vi "TalonWorking.vi"(1 "Name":string) -> (0 "Broken":bool)   [LabVIEW 2017]
uses:
  <vilib>/Rock Robotics/Network Tables/NT Write Boolean.vi
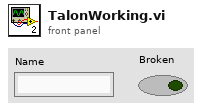
[diagram p1: front panel]
types:
  T1 = typedef "WPI_MotorControlDeviceRef.ctl" = cluster{"DeviceStatus":errorcluster, "Type":T2, "PWM":cluster{"PWM Channel":T3, "DeadBand":T4}, "CAN":cluster{"Device Number":u8, "SetOutput VI Ref":variant, "GetOutput VI Ref":variant, "Enable VI Ref":variant, "Disable VI Ref":variant, "Data":variant}, "Invert":bool, "DIO PWM":cluster{"PWM \"Enable\" Channel":T3, "DIOChannel":T5, "PWM Rate":dbl}}
  T2 = typedef "WPI_MotorControlType.ctl" = enum16{"PWM", "CAN", "DIO PWM"}
  T3 = typedef "FPGA_DIOPWMChannel.ctl" = enum8{"PWM 0", "PWM 1", "PWM 2", "PWM 3", "PWM 4", "PWM 5", "PWM 6", "PWM 7", "PWM 8", "PWM 9", "PWM MXP 0", "PWM MXP 1", "PWM MXP 2", "PWM MXP 3", "PWM MXP 4", "PWM MXP 5", "PWM MXP 6", "PWM MXP 7", "PWM MXP 8", "PWM MXP 9", "Invalid"}
  T4 = typedef "WPI_PWMDeadband.ctl" = cluster{"Name":string, "maxPositivePwm":i32, "minPositivePwm":i32, "centerPwm":i32, "maxNegativePwm":i32, "minNegativePwm":i32, "angularRange":u16}
  T5 = typedef "FPGA_DIOChannel.ctl" = enum8{"DIO 0", "DIO 1", "DIO 2", "DIO 3", "DIO 4", "DIO 5", "DIO 6", "DIO 7", "DIO 8", "DIO 9", "DIO MXP 0", "DIO MXP 1", "DIO MXP 2", "DIO MXP 3", "DIO MXP 4", "DIO MXP 5", "DIO MXP 6", "DIO MXP 7", "DIO MXP 8", "DIO MXP 9", "DIO MXP 10", "DIO MXP 11", "DIO MXP 12", "DIO MXP 13", "DIO MXP 14", "DIO MXP 15", "SPI Port CS1", "SPI Port CS2", "SPI Port CS3", "SPI Port MISO", "SPI Port MOSI", "Invalid"}
  T6 = cluster{"Under Voltage":bool, "Forward Limit Switch":bool, "Reverse Limit Switch":bool, "Forward Soft Limit":bool, "Reverse Soft Limit":bool, "Hardware Failure":bool, "Reset During Enable":bool, "Sensor Overflow":bool, "Sensor Out of Phase":bool, "Hardware ESD Reset":bool, "Remote Loss of Signal":bool}
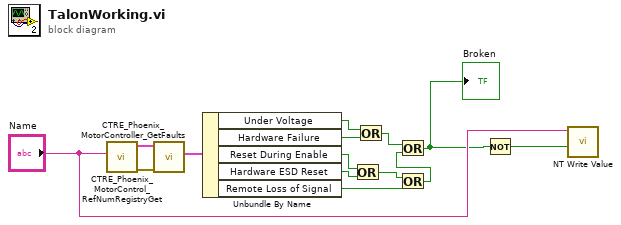
[diagram p0: block diagram]
diagram:
  n1 = call "CTRE_Phoenix_MotorControl_RefNumRegistryGet.vi"("refnum name"="Name") -> ("error out"=w5:errorcluster, "PhoenixMotorControlDevRef"=w4:T1)  [unwired: 9 in]
  n2 = call "CTRE_Phoenix_MotorController_GetFaults.vi"("error in"=w5, "PhoenixMotorControlDevRef"=w4) -> ("Faults"=w14:T6)  [unwired: 7 in, 2 out]
  n3 = Unbundle By Name(w14) -> ("Under Voltage"=w13:bool, "Hardware Failure"=w12:bool, "Reset During Enable"=w11:bool, "Hardware ESD Reset"=w10:bool, "Remote Loss of Signal"=w9:bool)
  n4 = Or(x=w11, y=w10) -> (x .or. y?=w8:bool)
  n5 = Or(x=w13, y=w12) -> (x .or. y?=w7:bool)
  n6 = Or(x=w8, y=w9) -> (x .or. y?=w6:bool)
  n7 = Or(x=w7, y=w6) -> (x .or. y?=w1:bool)
  "Broken" <- w1
  n8 = Not(x=w1) -> (.not. x?=w3:bool)
  n9 = call-poly <vilib>:"NT Write Value.vi"("Boolean"=w3, "Name"="Name") -> ()  [unwired: 9 in, 1 out]
